vi "Run Python Script.vi"(7 "Server Alias":string, 8 "error in (no error)":errorcluster, 10 "Script Arguments (Optional)":string[](array[string]), 11 "Absolute Python Script Path":path) -> (0 "error out":errorcluster)   [LabVIEW 2013, in "TS.lvlib"]
doc: "This VI runs a Python script by packaging the script path and optional arguments into the Data array/list, and sending the command \"run_script\".s"
uses:
  TS.lvlib
  LabVIEW Python Connector Message.ctl
  <vilib>/ErrorRing/Error Ring.xnode
  <vilib>/Utility/error.llb/Error Cluster From Error Code.vi
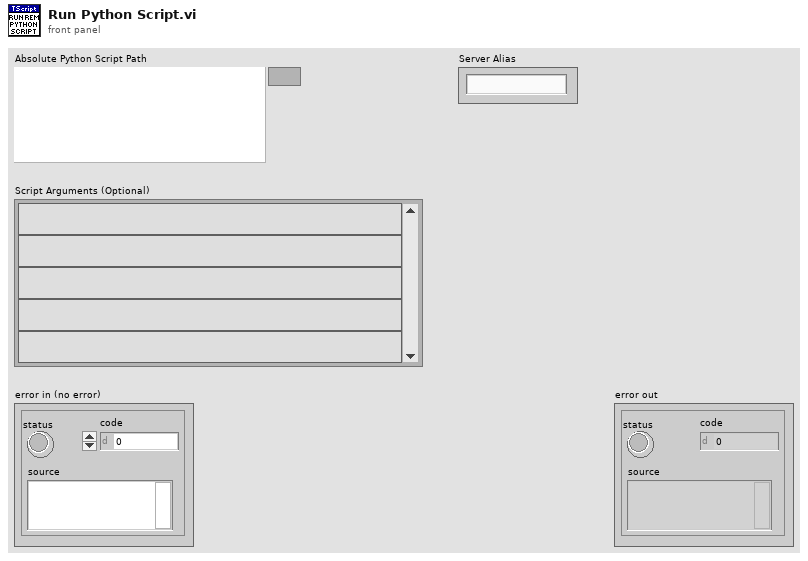
[diagram p1: front panel]
types:
  T1 = enum16{"open", "replace", "create", "open or create", "replace or create", "replace or create with confirmation"}
  T2 = typedef "TS.lvlib/LabVIEW Python Connector Message.ctl" = cluster{"Command":string, "Data":string[], "Script ID":i64, "LabVIEW Server ID":string, "Python Message ID":i32}
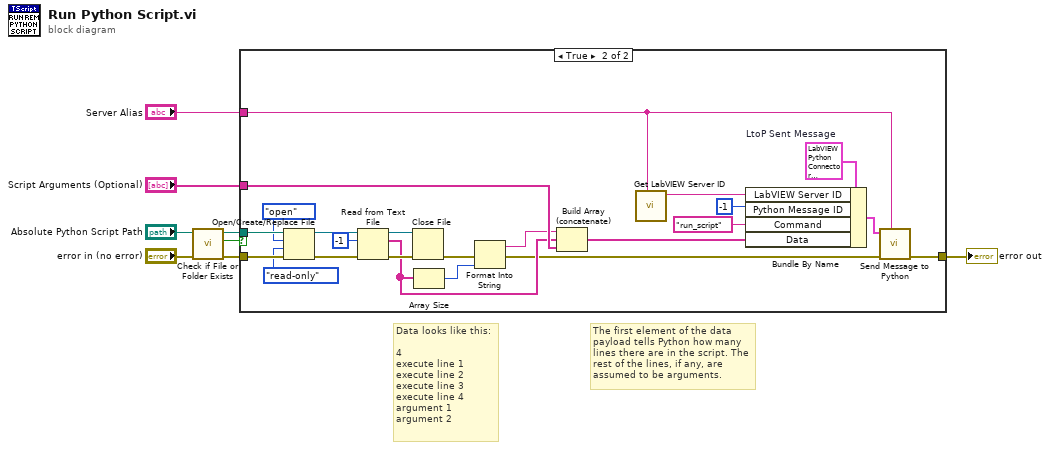
[diagram p0: block diagram]
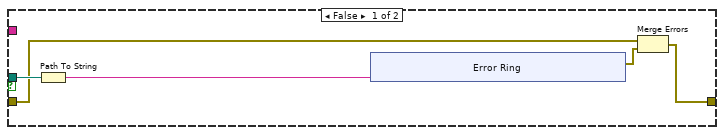
[diagram p2: hidden frame]
diagram:
  # "The first element of the data\npayload tells Python how many\nlines there are in the script. The\nrest of the lines, if any, are \nassumed to be arguments."
  # "Data looks like this:\n\n4\nexecute line 1\nexecute line 2\nexecute line 3\nexecute line 4\nargument 1\nargument 2"
  n1 = call <vilib>:"Check if File or Folder Exists.vi"("error in (no error)"="error in (no error)", "path"="Absolute Python Script Path") -> ("error out"=w5:errorcluster, "file or folder exists?"=w4:bool, "dup path"=w3:path)  [unwired: 7 in]
  n2 = case shown="True" w4 {
    tunnel: [w9 w43] -> w8
    tunnel: w5 -> [w10 w34]
    tunnel: w3 -> [w13 w33]
    tunnel: "Script Arguments (Optional)" -> [_ w38]
    tunnel: "Server Alias" -> [_ w35]
    frame False {
      n3 = Path To String(path=w13) -> (string=w12:string)
      n4 = xnode "Error Ring"("parameter 0"=w12) -> ("error out"=w11:errorcluster)
      n5 = Merge Errors(w10, w11) -> (w9:errorcluster)
    }
    frame True {
      w42 = T2 {"Command"="run_customer_script", "Data"=[], "Script ID"=0, "LabVIEW Server ID"="zxcvbnm,", "Python Message ID"=0}  # LtoP Sent Message
      n6 = Open/Create/Replace File(file path (use dialog)=w33, error in=w34, operation (0:open)=T1."open", access (0:read/write)=enum16{"read/write", "read-only", "write-only"}."read-only") -> (refnum out=w29:refnum<file>, error out=w30:errorcluster)  [unwired: 2 in, 1 out]
      n7 = Read from Text File(file (use dialog)=w29, count=-1, error in=w30) -> (refnum out=w26:refnum<file>, text=w22:string[], error out=w27:errorcluster)  [unwired: 1 in, 1 out]
      n8 = Close File(refnum=w26, error in=w27) -> (error out=w25:errorcluster)  [unwired: 1 out]
      n9 = Array Size(array=w22) -> (size(s)=w24:i32)
      n10 = Format Into String(error in=w25, w24) -> (resulting string=w23:string, error out=w21:errorcluster)  [unwired: 2 in]
      n11 = Build Array (concatenate)(w23, w22, w38) -> (w41:string[])
      n12 = call "Get LabVIEW Server ID.vi"("Server Alias"=w35) -> ("LabVIEW Server ID"=w36:string)  [unwired: 9 in, 1 out]
      n13 = Bundle By Name(cluster=w42, "LabVIEW Server ID"=w36, "Python Message ID"=-1, "Command"="run_script", "Data"=w41) -> (w39:T2)
      n14 = call "Send Message to Python.vi"("Server Alias"=w35, "error in (no error)"=w21, "Message"=w39) -> ("error out"=w43:errorcluster)  [unwired: 8 in]
    }
  }
  "error out" <- w8
